vi "GetType.vi"(8 "error in (no error)":errorcluster, 11 "Initialize Device Msg":refnum<class "Initialize Device Msg.lvclass">) -> (0 "error out":errorcluster, 2 "Data Sample":variant, 3 "Initialize Device Msg":refnum<class "Initialize Device Msg.lvclass">)   [LabVIEW 2015, in "CS++DeviceActor.lvlib" / "Initialize Device Msg.lvclass"]
doc: "This VI delivers a sample of the data type format the message expects."
uses:
  Initialize Device Msg.lvclass
  Initialize Device Msg.lvclass/Initialize Device Msg.ctl
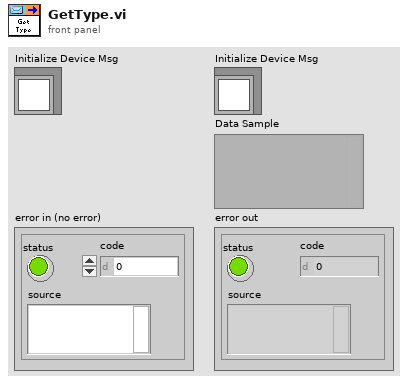
[diagram p1: front panel]
types:
  T1 = cluster{"Resource Name":string, "Reset (F)":bool}
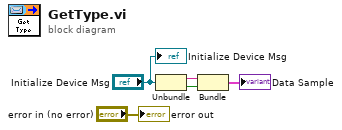
[diagram p0: block diagram]
diagram:
  n1 = Unbundle("Initialize Device Msg") -> (w2:string, w1:bool)
  n2 = Bundle("Resource Name"=w2, "Reset (F)"=w1) -> (→"Data Sample":T1)  [unwired: 1 in]
  "error out" <- "error in (no error)"
  "Initialize Device Msg" <- "Initialize Device Msg"
